vi "CallbackOnLoadUI.vi"(8 "error in":errorcluster, 11 "node":refnum<data-value>) -> (0 "error out":errorcluster)   [LabVIEW 2013, in "NISE_CEF_Node.lvclass"]
uses:
  NISE_CEF_Node.lvclass
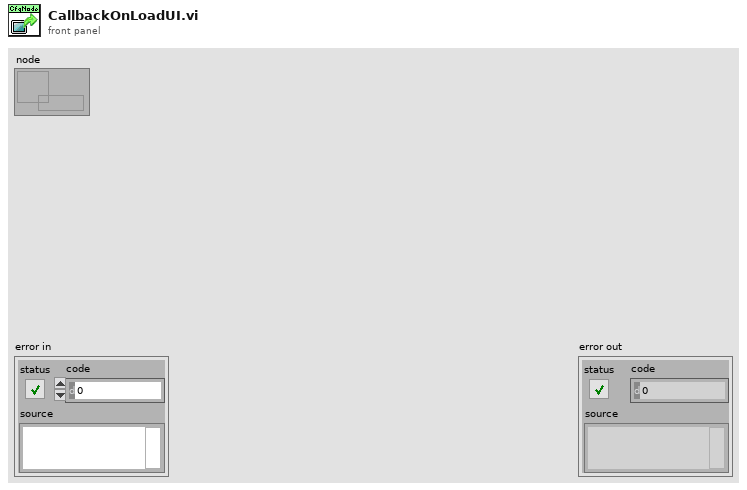
[diagram p1: front panel]
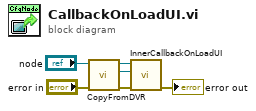
[diagram p0: block diagram]
diagram:
  n1 = call "CopyFromDVR.vi"("error in"="error in", "node in"="node") -> ("error out"=w4:errorcluster, "NISE_CEF_Node out"=w2:refnum<class "NISE_CEF_Node.lvclass">, "node out"=w1:refnum<data-value>)  [unwired: 7 in]
  n2 = call-dynamic "InnerCallbackOnLoadUI.vi"("error in"=w4, "node (for type)"=w2, "node reference"=w1) -> ("error out"=→"error out":errorcluster)  [unwired: 8 in]
